vi "Spectrograph_cancelCallback_command_enable.vi"(8 "error in (no error)":errorcluster) -> (0 "error out":errorcluster, 3 "function return":i32)   [LabVIEW 2016, in "SALLV_Spectrograph.lvlib"]
doc: "int Spectrograph_shm_cancelCallback_command_enableLV();"
uses:
  SALLV_Spectrograph.lvlib
  SALLV_Spectrograph.so
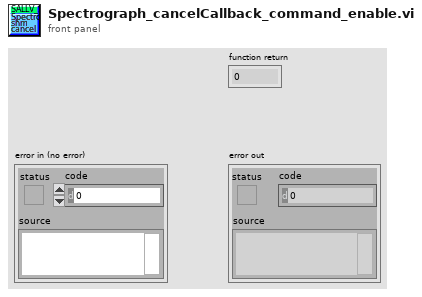
[diagram p1: front panel]
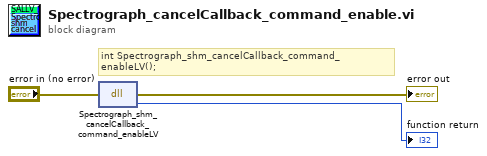
[diagram p0: block diagram]
diagram:
  # "int Spectrograph_shm_cancelCallback_command_enableLV();"
  n1 = dll-call lib="home/harini/TCS/SALLV_Spectrograph/SALLV_Spectrograph.*" fn="Spectrograph_shm_cancelCallback_command_enableLV"(error in="error in (no error)") -> (error out=→"error out":errorcluster, →"function return":i32)  [unwired: 2 in, 1 out]
